vi "Tektronix 7000 Series Transfer Current Waveform To File.vi"() -> ()   [LabVIEW 2015]
doc: "This example illustrates how to transfer the current waveform to the file on an oscilloscope. You can use the <B> Read Waveform from File Interactive Example.vi</B> or <B> Read Waveform From File Example.vi</B> to read the waveform from the file."
uses:
  <instrlib>/Tektronix 7000 Series/Public/Data/Low Level/Fetch (Waveform To File).vi
  <instrlib>/Tektronix 7000 Series/Tektronix 7000 Series.lvlib
panel:
  in  "Maximum Time (200000ms)":u32=200000
  in  "Channel (0: Channel 1)":u16(ring) format="%#_5f" items=["Channel 1", "Channel 2", "Channel 3", "Channel 4", "Math 1", "Math 2", "Math 3", "Math 4", "Reference 1", "Reference 2", "Reference 3", "Reference 4"]
  in  "Filename (C:\\data.txt)":path=path "C:/data.txt"
  in  "VISA resource name":refnum<visa-resource-name>
  # "(c) 2006 - 2016 National Instruments Corporation.  ALL RIGHTS RESERVED."
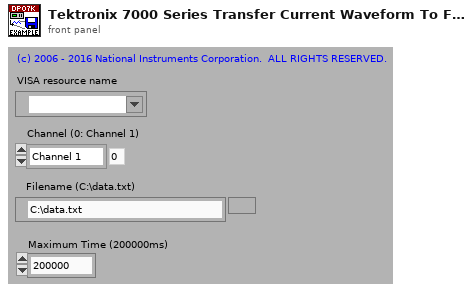
[diagram p1: front panel]
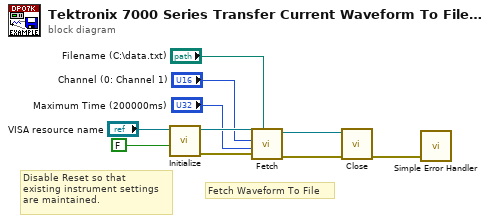
[diagram p0: block diagram]
diagram:
  # "Fetch Waveform To File"
  # "Disable Reset so that \nexisting instrument settings are maintained."
  n1 = call <instrlib>:"Initialize.vi"("Reset? ( Yes)"=FALSE, "VISA resource name"="VISA resource name") -> ("error out"=w10:errorcluster, "VISA resource name out"=w9:refnum<visa-resource-name>)  [unwired: 8 in]
  n2 = call-poly <instrlib>:"Fetch.vi"("Filename (C:\\data.txt)"="Filename (C:\\data.txt)", "error in (no error)"=w10, "Maximum Time (200000ms)"="Maximum Time (200000ms)", "Channel (0:Channel1)"="Channel (0: Channel 1)", "VISA resource name"=w9) -> ("error out"=w7:errorcluster, "VISA resource name out"=w8:refnum<visa-resource-name>)  [unwired: 5 in]
  n3 = call <instrlib>:"Close.vi"("error in (no error)"=w7, "VISA resource name"=w8) -> ("error out"=w6:errorcluster)  [unwired: 9 in]
  n4 = call <vilib>:"Simple Error Handler.vi"("error in (no error)"=w6) -> ()  [unwired: 4 in, 5 out]
